vi "Logger.Variant.Write.vi"(8 "error in (no error)":errorcluster, 10 "VariantSets":T1={"State"=enum."Init", "ImgPath"=path "", "WabcoPlate"="", "WabcoProduct"="", "ClientProduct"="", "ClientPlate"="", "TotalQuantity"=0, "OrderQuantity"=0, "Serial"=0, "Wabco"={"LaserJob"="", "AdditionalTxt"="037", "FactoryCode"="", "RevID"=0, "ForkID"=0, "FailuresLimit"=0, "GlobalCnt"=0, "ScannerProgram"=0, "SerialFormat"=enum."6 dig", "CoordA"={"X"=0.0, "Y"=0.0, "Angle"=0.0}, "CoordB"={"X"=0.0, "Y"=0.0, "Angle"=0.0}, "DMCconfig"=0, "CVX_Program"=0}, "Client"={"LaserJob"="", "AdditionalTxt"="", "FactoryCode"="037", "RevID"=0, "ForkID"=0, "FailuresLimit"=0, "GlobalCnt"=0, "ScannerProgram"=0, "SerialFormat"=enum."6 dig", "CoordA"={"X"=0.0, "Y"=0.0, "Angle"=0.0}, "CoordB"={"X"=0.0, "Y"=0.0, "Angle"=0.0}, "DMCconfig"=0, "CVX_Program"=0}}) -> (0 "error out":errorcluster)   [LabVIEW 2016]
uses:
  Logger.Variant.Sets.ctl
  Station/Station.Changeover.State.vi
  Station/Station.Plate.Properties.ctl
  Sequence/Sequence.Code.SerialFormat.ctl
  Drivers/V7310/LowLevel/V7310.Job.Sets.ctl
  Global/ApplicationGlobal.vi
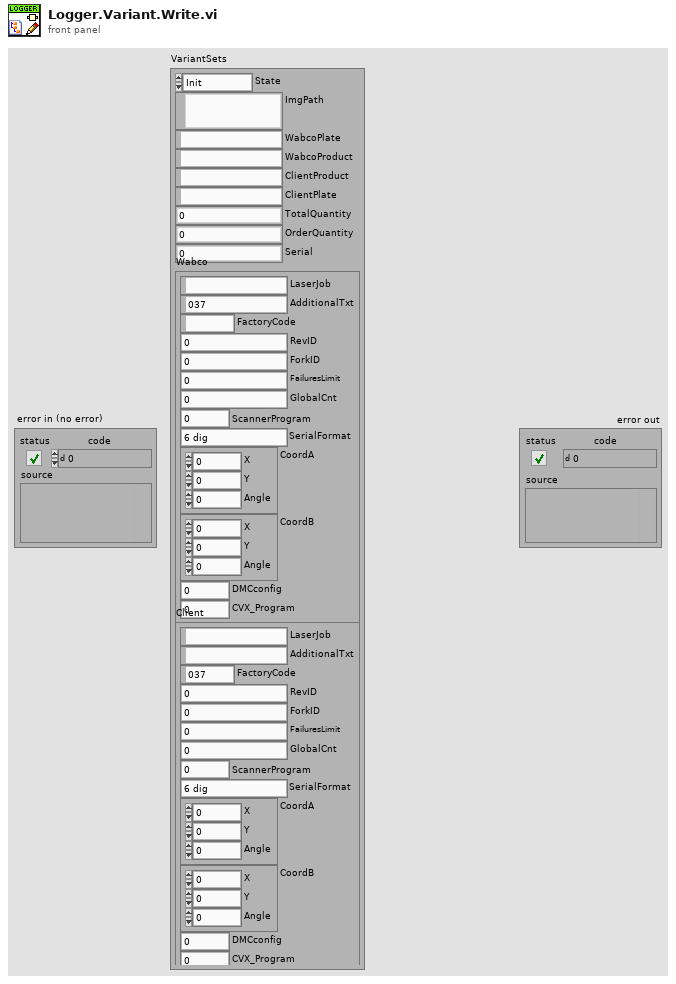
[diagram p1: front panel]
types:
  T1 = typedef "Logger.Variant.Sets.ctl" = cluster{"State":T2, "ImgPath":path, "WabcoPlate":string, "WabcoProduct":string, "ClientProduct":string, "ClientPlate":string, "TotalQuantity":u16, "OrderQuantity":u16, "Serial":i32, "Wabco":T3, "Client":T3}
  T2 = typedef "Station.Changeover.State.vi" = enum16{"Init", "Scaning", "NOK", "Wait for ack", "Ready"}
  T3 = typedef "Station.Plate.Properties.ctl" = cluster{"LaserJob":string, "AdditionalTxt":string, "FactoryCode":string, "RevID":u8, "ForkID":u8, "FailuresLimit":u16, "GlobalCnt":i32, "ScannerProgram":u8, "SerialFormat":T4, "CoordA":T5, "CoordB":T5, "DMCconfig":i32, "CVX_Program":u16}
  T4 = typedef "Sequence.Code.SerialFormat.ctl" = enum8{"", "6 dig", "7 dig"}
  T5 = typedef "V7310.Job.Sets.ctl" = cluster{"X":dbl, "Y":dbl, "Angle":dbl}
  T6 = cluster{"WabcoPlate":string, "WabcoProduct":string, "ClientProduct":string, "ClientPlate":string}
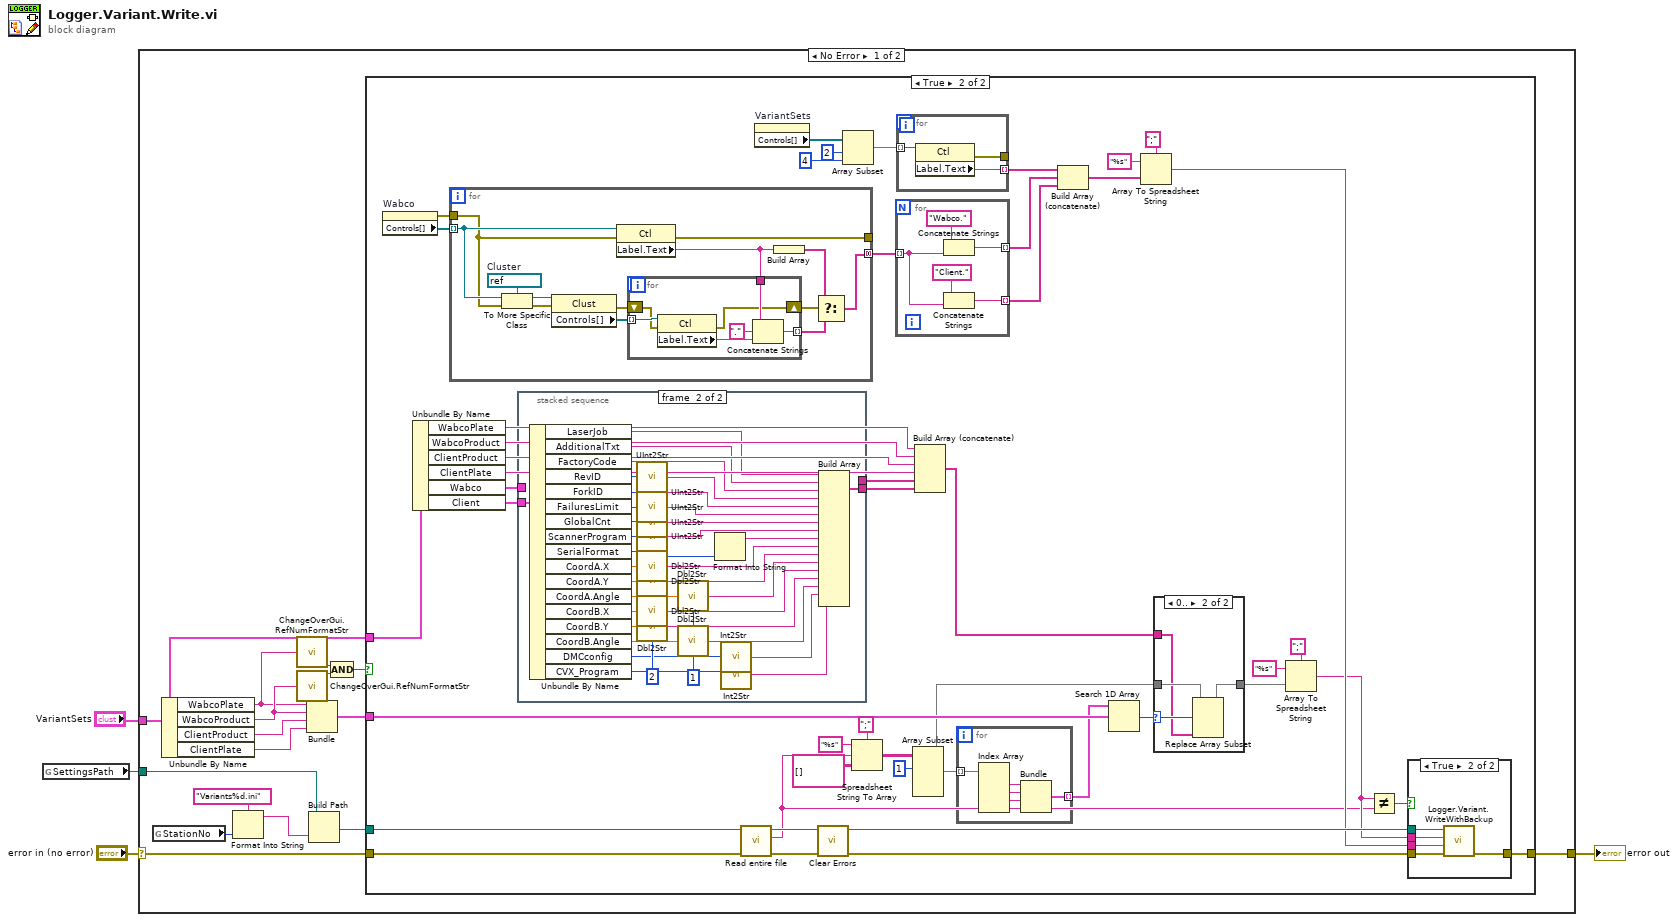
[diagram p0: block diagram]
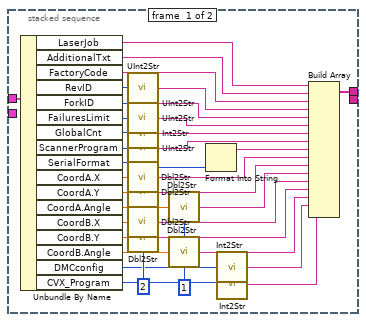
[diagram p4: hidden frame]
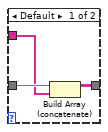
[diagram p5: hidden frame]
diagram:
  n1 = global read "ApplicationGlobal.vi" "SettingsPath"() -> (w2:path)
  n2 = case shown="No Error" "error in (no error)" {
    selector: "error in (no error)" -> [w20 w183]
    tunnel: [w19 w183] -> w3
    tunnel: w2 -> [w8 _]
    tunnel: "VariantSets" -> [w10 _]
    frame No Error {
      n3 = global read "ApplicationGlobal.vi" "StationNo"() -> (w5:i32)
      n4 = Unbundle By Name(w10) -> ("WabcoPlate"=w15:string, "WabcoProduct"=w16:string, "ClientProduct"=w17:string, "ClientPlate"=w9:string)
      n5 = Format Into String(format string="Variants%d.ini", w5) -> (resulting string=w6:string)  [unwired: 2 in, 1 out]
      n6 = call "ChangeOverGui.RefNumFormatStr.vi"("RefNum in"=w15) -> ("RefNum format ok?"=w14:bool)  [unwired: 2 out]
      n7 = call "ChangeOverGui.RefNumFormatStr.vi"("RefNum in"=w16) -> ("RefNum format ok?"=w13:bool)  [unwired: 2 out]
      n8 = Bundle("WabcoPlate"=w15, "WabcoProduct"=w16, "ClientProduct"=w17, "ClientPlate"=w9) -> (w11:T6)  [unwired: 1 in]
      n9 = Build Path(base path=w8, name or relative path=w6) -> (appended path=w18:path)
      n10 = Compound Arithmetic op=AND(w14, w13) -> (w12:bool)
      n11 = case shown="True" w12 {
        tunnel: w20 -> [w21 w65]
        tunnel: [w21 w56] -> w19
        tunnel: w18 -> [_ w51]
        tunnel: w11 -> [_ w60]
        tunnel: w10 -> [_ w44]
        frame False {
        }
        frame True {
          n12 = property on="Wabco" class="Clust (strict)"() -> (error out=w26:errorcluster, "Controls[]"=w27:refnum<vi>[])  [unwired: 2 in, 1 out]
          n13 = Unbundle By Name(w44) -> ("WabcoPlate"=w34:string, "WabcoProduct"=w33:string, "ClientProduct"=w32:string, "ClientPlate"=w31:string, "Wabco"=w40:T3, "Client"=w37:T3)
          n14 = for {
            tunnel: w27 -> [w85] mode=indexing
            tunnel: [w78] -> w30 mode=concatenating
            tunnel: [w89] -> _
            tunnel: w26 -> [w77]
            w87 = refnum<vi> refnum  # Cluster
            n15 = To More Specific Class(target class=w87, reference=w85, error in=w77) -> (specific class reference=w86:refnum<vi>, error out=w88:errorcluster)
            n16 = property class="Clust"(reference=w86, error in=w88) -> (error out=w83:errorcluster, "Controls[]"=w84:refnum<vi>[])  [unwired: 1 out]
            n17 = property class="Ctl"(reference=w85, error in=w77) -> (error out=w89:errorcluster, "Label.Text"=w82:string)  [unwired: 1 out]
            n18 = for {
              tunnel: w84 -> [w96] mode=indexing
              tunnel: [w93] -> w79 mode=indexing
              tunnel: w82 -> [w92]
              shift-right: [w90] -> w81
              shift-left: w83 -> [w95]
              n19 = property class="Ctl"(reference=w96, error in=w95) -> (error out=w90:errorcluster, "Label.Text"=w94:string)  [unwired: 1 out]
              n20 = Concatenate Strings(w92, "." ("string"), w94) -> (w93:string)
            }
            n21 = Build Array(w82) -> (w80:string[])
            n22 = Select(t=w80, s=w81, f=w79) -> (s? t:f=w78:string[])
          }
          n23 = stacked-sequence {
            tunnel: w40 -> [w131 _]
            tunnel: [w103 _] -> w39
            tunnel: [_ w139] -> w38
            tunnel: w37 -> [_ w138]
            frame #0 {
              w129 = i16 2 ("precision (6)")
              w130 = i16 1 ("precision (6)")
              n24 = Unbundle By Name(w131) -> ("LaserJob"=w104:string, "AdditionalTxt"=w105:string, "FactoryCode"=w106:string, "RevID"=w113:u8, "ForkID"=w114:u8, "FailuresLimit"=w112:u16, "GlobalCnt"=w111:i32, "ScannerProgram"=w100:u8, "SerialFormat"=w116:T4, "CoordA.X"=w128:dbl, "CoordA.Y"=w127:dbl, "CoordA.Angle"=w126:dbl, "CoordB.X"=w125:dbl, "CoordB.Y"=w124:dbl, "CoordB.Angle"=w123:dbl, "DMCconfig"=w102:i32, "CVX_Program"=w98:u16)
              n25 = call "UInt2Str.vi"("Numeric"=w113) -> ("string"=w107:string)
              n26 = call "UInt2Str.vi"("Numeric"=w114) -> ("string"=w108:string)
              n27 = call "UInt2Str.vi"("Numeric"=w112) -> ("string"=w109:string)
              n28 = call "Int2Str.vi"("Numeric"=w111) -> ("string"=w110:string)
              n29 = call "UInt2Str.vi"("Numeric"=w100) -> ("string"=w99:string)
              n30 = call "Dbl2Str.vi"("Numeric"=w128, "precision (6)"=w129) -> ("string"=w117:string)
              n31 = call "Dbl2Str.vi"("Numeric"=w127, "precision (6)"=w129) -> ("string"=w118:string)
              n32 = call "Dbl2Str.vi"("Numeric"=w125, "precision (6)"=w129) -> ("string"=w120:string)
              n33 = call "Dbl2Str.vi"("Numeric"=w124, "precision (6)"=w129) -> ("string"=w121:string)
              n34 = call "Dbl2Str.vi"("Numeric"=w126, "precision (6)"=w130) -> ("string"=w119:string)
              n35 = call "Dbl2Str.vi"("Numeric"=w123, "precision (6)"=w130) -> ("string"=w122:string)
              n36 = Format Into String(w116) -> (resulting string=w115:string)  [unwired: 3 in, 1 out]
              n37 = call "Int2Str.vi"("Numeric"=w102) -> ("string"=w101:string)
              n38 = call "Int2Str.vi"("Numeric"=w98) -> ("string"=w97:string)
              n39 = Build Array(w104, w105, w106, w107, w108, w109, w110, w99, w115, w117, w118, w119, w120, w121, w122, w101, w97) -> (w103:string[])
            }
            frame #1 {
              w165 = i16 2 ("precision (6)")
              w166 = i16 1 ("precision (6)")
              n40 = Unbundle By Name(w138) -> ("LaserJob"=w140:string, "AdditionalTxt"=w141:string, "FactoryCode"=w142:string, "RevID"=w149:u8, "ForkID"=w150:u8, "FailuresLimit"=w148:u16, "GlobalCnt"=w147:i32, "ScannerProgram"=w135:u8, "SerialFormat"=w152:T4, "CoordA.X"=w164:dbl, "CoordA.Y"=w163:dbl, "CoordA.Angle"=w162:dbl, "CoordB.X"=w161:dbl, "CoordB.Y"=w160:dbl, "CoordB.Angle"=w159:dbl, "DMCconfig"=w137:i32, "CVX_Program"=w133:u16)
              n41 = call "UInt2Str.vi"("Numeric"=w149) -> ("string"=w143:string)
              n42 = call "UInt2Str.vi"("Numeric"=w150) -> ("string"=w144:string)
              n43 = call "UInt2Str.vi"("Numeric"=w148) -> ("string"=w145:string)
              n44 = call "UInt2Str.vi"("Numeric"=w147) -> ("string"=w146:string)
              n45 = call "UInt2Str.vi"("Numeric"=w135) -> ("string"=w134:string)
              n46 = call "Dbl2Str.vi"("Numeric"=w164, "precision (6)"=w165) -> ("string"=w153:string)
              n47 = call "Dbl2Str.vi"("Numeric"=w163, "precision (6)"=w165) -> ("string"=w154:string)
              n48 = call "Dbl2Str.vi"("Numeric"=w161, "precision (6)"=w165) -> ("string"=w156:string)
              n49 = call "Dbl2Str.vi"("Numeric"=w160, "precision (6)"=w165) -> ("string"=w157:string)
              n50 = call "Dbl2Str.vi"("Numeric"=w162, "precision (6)"=w166) -> ("string"=w155:string)
              n51 = call "Dbl2Str.vi"("Numeric"=w159, "precision (6)"=w166) -> ("string"=w158:string)
              n52 = Format Into String(w152) -> (resulting string=w151:string)  [unwired: 3 in, 1 out]
              n53 = call "Int2Str.vi"("Numeric"=w137) -> ("string"=w136:string)
              n54 = call "Int2Str.vi"("Numeric"=w133) -> ("string"=w132:string)
              n55 = Build Array(w140, w141, w142, w143, w144, w145, w146, w134, w151, w153, w154, w155, w156, w157, w158, w136, w132) -> (w139:string[])
            }
          }
          n56 = call "Read entire file.vi"("error in"=w65, "file"=w51) -> ("error out"=w55:errorcluster, "contents"=w23:string)  [unwired: 4 in]
          n57 = property on="VariantSets" class="Clust (strict)"() -> ("Controls[]"=w42:refnum<vi>[])  [unwired: 2 in, 2 out]
          n58 = call <vilib>:"Clear Errors.vi"("error in (no error)"=w55) -> ("error out"=w47:errorcluster)  [unwired: 5 in, 1 out]
          n59 = Array Subset(array=w42, index=2, length=4) -> (w36:refnum<vi>[])
          n60 = Spreadsheet String To Array(delimiter (Tab)=";", format string="%s", spreadsheet string=w23, array type (2D Dbl)=string[][] []) -> (array=w57:string[][])
          n61 = for {
            tunnel: w30 -> [w73] mode=indexing
            tunnel: [w75] -> w29 mode=indexing
            tunnel: [w72] -> w28 mode=indexing
            n62 = Concatenate Strings("Wabco." ("string"), w73) -> (w75:string)
            n63 = Concatenate Strings("Client." ("string"), w73) -> (w72:string)
          }
          n64 = for {
            tunnel: w36 -> [w182] mode=indexing
            tunnel: [w181] -> w48 mode=indexing
            tunnel: [w180] -> _
            n65 = property class="Ctl"(reference=w182) -> (error out=w180:errorcluster, "Label.Text"=w181:string)  [unwired: 1 in, 1 out]
          }
          n66 = Array Subset(array=w57, index (row)=1 ("index")) -> (w46:string[][])  [unwired: 3 in]
          n67 = Build Array (concatenate)(w34, w33, w32, w31, w39, w38) -> (w41:string[])
          n68 = for {
            tunnel: w46 -> [w168] mode=indexing
            tunnel: [w169] -> w59 mode=indexing
            n69 = Index Array(array=w168) -> (element #1=w172:string, element #2=w171:string, element #3=w170:string, element #4=w167:string)  [unwired: 4 in]
            n70 = Bundle(w172, w171, w170, w167) -> (w169:cluster{string, string, string, string})  [unwired: 1 in]
          }
          n71 = Build Array (concatenate)(w48, w29, w28) -> (w35:string[])
          n72 = Search 1D Array(1D array=w59, element=w60) -> (index of element=w58:i32)  [unwired: 1 in]
          n73 = Array To Spreadsheet String(delimiter (Tab)=";", array=w35, 3:"%s" ("format string")) -> (spreadsheet string=w25:string)
          n74 = case shown="0.." w58 {
            selector: w58 -> [_ w177]
            tunnel: w46 -> [w175 w179]
            tunnel: [w173 w178] -> w54
            tunnel: w41 -> [w174 w176]
            frame Default {
              n75 = Build Array (concatenate)(w175, w174) -> (w173:string[][])
            }
            frame 0.. {
              n76 = Replace Array Subset(array=w179, new element=w176, index (row)=w177) -> (w178:string[][])  [unwired: 1 in]
            }
          }
          n77 = Array To Spreadsheet String(delimiter (Tab)=";", array=w54, 3:"%s" ("format string")) -> (spreadsheet string=w24:string)
          n78 = Not Equal?(x=w24, y=w23) -> (x != y?=w22:bool)
          n79 = case shown="True" w22 {
            tunnel: [w66 w71] -> w56
            tunnel: w51 -> [_ w70]
            tunnel: w47 -> [w66 w69]
            tunnel: w25 -> [_ w68]
            tunnel: w24 -> [_ w67]
            frame False {
            }
            frame True {
              n80 = call "Logger.Variant.WriteWithBackup.vi"("error in"=w69, "header"=w68, "addition"=w67, "file"=w70) -> ("error out"=w71:errorcluster)  [unwired: 7 in]
            }
          }
        }
      }
    }
    frame Error {
    }
  }
  "error out" <- w3
